vi "simple DAQ test.vi"() -> ()   [LabVIEW 2011]
panel:
  out "Numeric":i32
  in  "stop":bool
  out "Filename Out":path
  in  "Record Data":bool
  in  "error in":errorcluster
  in  "File Name":path=path "C:/Documents and Settings/QIM/My Documents/LabVIEW Data/111016-discord-gain9-seed40-3/ele-0000mV-d0150mV-g9-s40.lvm"
  out "error out":errorcluster
  out "Saving Data":bool
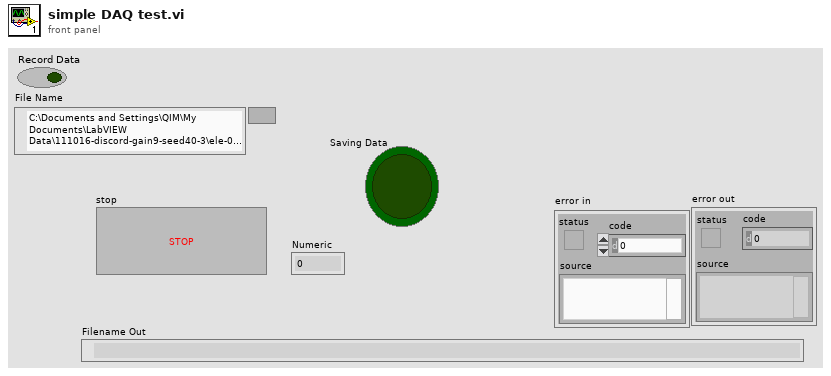
[diagram p1: front panel]
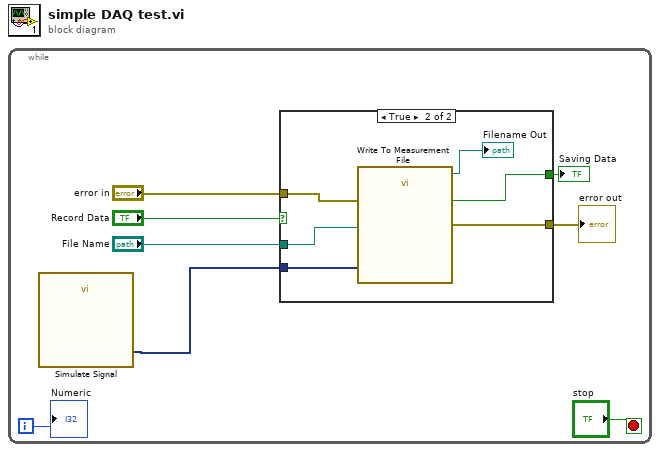
[diagram p0: block diagram]
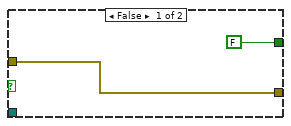
[diagram p2: hidden frame]
diagram:
  n1 = while {
    i -> [w1]
    stop <- "stop" stop-if-true
    n2 = call "Simulate Signal"() -> ("Sine"=w3:dynamicdata)  [unwired: 14 in, 1 out]
    n3 = case shown="True" "Record Data" {
      tunnel: "error in" -> [w10 w16]
      tunnel: "File Name" -> [_ w15]
      tunnel: [w10 w14] -> w7
      tunnel: [FALSE ("Saving Data") w13] -> w8
      tunnel: w3 -> [_ w11]
      frame False {
      }
      frame True {
        n4 = call "Write To Measurement File"("Signals"=w11, "error in (no error)"=w16, "Filename"=w15) -> ("Filename Out"=→"Filename Out":path, "Saving Data"=w13:bool, "error out"=w14:errorcluster)  [unwired: 14 in]
      }
    }
    "error out" <- w7
    "Saving Data" <- w8
    "Numeric" <- w1
  }
